vi "Browser.vi"(11 "html":string="<html><head><title>Rogers Camera Code</title></head><body><p>Rogers Camera</p><p>You accessed path: /</p></body></html>\r\n") -> (3 "2D Picture":picture)   [LabVIEW 2020]
panel:
  in  "Body":T1={"Font Name:"="Arial", "Size"=12, "Strikeout?"=FALSE, "Italic?"=FALSE, "Underline?"=FALSE, "Outline?"=FALSE, "Shadow?"=FALSE, "Bold?"=FALSE}
  in  "Title":T1={"Font Name:"="Arial", "Size"=12, "Strikeout?"=FALSE, "Italic?"=FALSE, "Underline?"=TRUE, "Outline?"=FALSE, "Shadow?"=FALSE, "Bold?"=TRUE}
  out "body fixed":string="Rogers Camera\n\nYou accessed path: /\n\n"
  out "title":string="Rogers Camera Code"
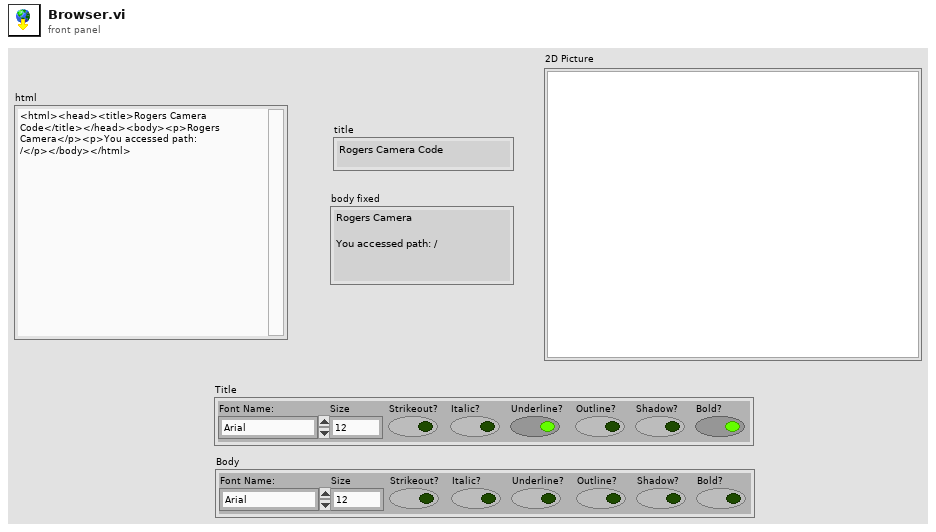
[diagram p1: front panel]
types:
  T1 = cluster{"Font Name:":string, "Size":i16, "Strikeout?":bool, "Italic?":bool, "Underline?":bool, "Outline?":bool, "Shadow?":bool, "Bold?":bool}
  T2 = cluster{"horizontal":enum16{"left", "center", "right"}, "vertical":enum16{"top", "center", "bottom"}}
  T3 = enum16{"User-specified Font", "Application Font", "System Font", "Dialog Font"}
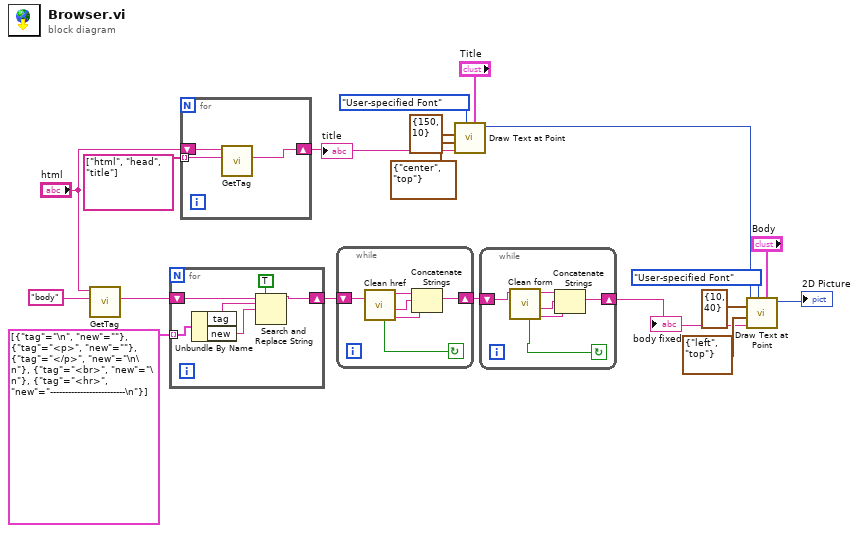
[diagram p0: block diagram]
diagram:
  n1 = call "GetTag.vi"("tag"="body", "String in"="html") -> ("body"=w16:string)  [unwired: 6 in, 3 out]
  n2 = for {
    shift-right: [w24] -> w3
    shift-left: w16 -> [w25]
    tunnel: cluster{"tag":string, "new":string}[] [{"tag"="\n", "new"=""}, {"tag"="<p>", "new"=""}, {"tag"="</p>", "new"="\n\n"}, {"tag"="<br>", "new"="\n"}, {"tag"="<hr>", "new"="-------------------------\n"}] -> [w23] mode=indexing
    n3 = Unbundle By Name(w23) -> ("tag"=w22:string, "new"=w21:string)
    n4 = Search and Replace String(replace all?=TRUE ("replace all? (F)"), input string=w25, search string=w22, replace string=w21) -> (result string=w24:string)  [unwired: 4 in, 3 out]
  }
  n5 = for {
    tunnel: string[] ["html", "head", "title"] -> [w28] mode=indexing
    shift-right: [w26] -> w10
    shift-left: "html" -> [w27]
    n6 = call "GetTag.vi"("tag"=w28, "String in"=w27) -> ("body"=w26:string)  [unwired: 6 in, 3 out]
  }
  "title" <- w10
  n7 = while {
    shift-right: [w29] -> w2
    shift-left: w3 -> [w34]
    stop <- w33 continue-if-true
    n8 = call "Clean href.vi"("html in"=w34) -> ("after hyperlink"=w30:string, "text"=w31:string, "before hyperlink"=w32:string, "Success?"=w33:bool)  [unwired: 6 in, 1 out]
    n9 = Concatenate Strings(w32, w31, w30) -> (w29:string)
  }
  n10 = call <vilib>:"Draw Text at Point.vi"("[user-specified font]"="Title", "desired font(Application)"=T3."User-specified Font", "text"=w10, "alignment(left, top)"=T2 {"horizontal"=enum."center", "vertical"=enum."top"}, "origin"=cluster{"x":i16, "y":i16} {"x"=150, "y"=10}) -> ("new picture"=w4:picture)  [unwired: 5 in, 1 out]
  n11 = while {
    shift-right: [w40] -> w1
    shift-left: w2 -> [w39]
    stop <- w36 continue-if-true
    n12 = call "Clean form.vi"("html in"=w39) -> ("after hyperlink"=w37:string, "text"=w35:string, "before hyperlink"=w38:string, "Success?"=w36:bool)  [unwired: 6 in, 1 out]
    n13 = Concatenate Strings(w38, w35, w37) -> (w40:string)
  }
  "body fixed" <- w1
  n14 = call <vilib>:"Draw Text at Point.vi"("[user-specified font]"="Body", "desired font(Application)"=T3."User-specified Font", "text"=w1, "alignment(left, top)"=T2 {"horizontal"=enum."left", "vertical"=enum."top"}, "origin"=cluster{"x":i16, "y":i16} {"x"=10, "y"=40}, "picture"=w4) -> ("new picture"=→"2D Picture":picture)  [unwired: 4 in, 1 out]
